vi "Measure.vi"(6 "error in (no error)":errorcluster, 9 "Tektronix PA1000 in":refnum<class "Tektronix PA1000.lvclass">) -> (0 "error out":errorcluster, 2 "Array of Measurement":dbl[](array[numeric]), 3 "Tektronix PA1000 out":refnum<class "Tektronix PA1000.lvclass">)   [LabVIEW 2014, in "Generic Power Analyzer.lvlib" / "Tektronix PA1000.lvlib" / "Tektronix PA1000.lvclass"]
uses:
  Tektronix PA1000.lvclass
  <instrlib>/Tektronix PA1000/Tektronix PA1000.lvlib
panel:
  out "VISA resource name":refnum<visa-resource-name>
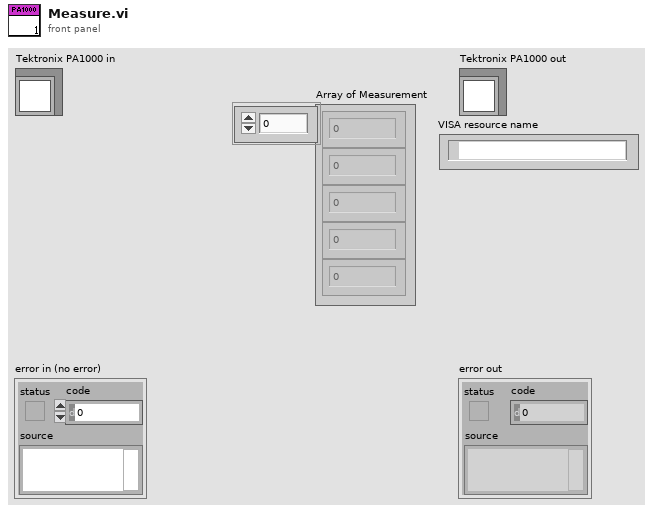
[diagram p1: front panel]
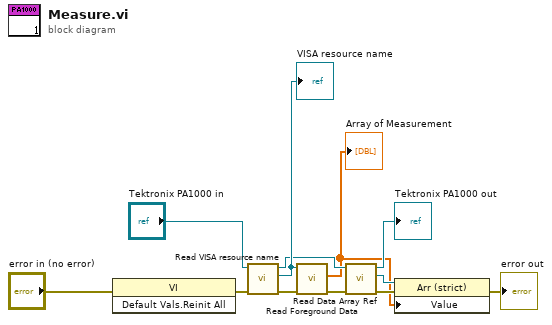
[diagram p0: block diagram]
diagram:
  n1 = invoke class="VI" method="Default Vals.Reinit All"(error in="error in (no error)") -> (error out=w1:errorcluster)  [unwired: 2 in, 2 out]
  n2 = call-dynamic "Read VISA resource name.vi"("error in (no error)"=w1, "Generic Instrument in"="Tektronix PA1000 in") -> ("error out"=w10:errorcluster, "VISA resource name"=w11:refnum<visa-resource-name>, "Generic Instrument out"=w9:refnum<class "Tektronix PA1000.lvclass">)  [unwired: 7 in]
  "VISA resource name" <- w11
  n3 = call <instrlib>:"Read Foreground Data.vi"("error in (no error)"=w10, "VISA resource name"=w11) -> ("error out"=w7:errorcluster, "Foreground Data"=w3:dbl[])  [unwired: 7 in, 1 out]
  "Array of Measurement" <- w3
  n4 = call-dynamic "Read Data Array Ref.vi"("error in (no error)"=w7, "Generic Instrument in"=w9) -> ("error out"=w5:errorcluster, "Data Array Ref"=w6:refnum<vi>, "Generic Instrument out"=→"Tektronix PA1000 out":refnum<class "Tektronix PA1000.lvclass">)  [unwired: 7 in]
  n5 = property class="Arr (strict)"(reference=w6, error in=w5, "Value"=w3) -> (error out=→"error out":errorcluster)  [unwired: 1 out]
